vi "Filter.vi"(8 "error in (no error)":errorcluster, 10 "Selected Runnables":string[](array[string]), 11 "LUnit Test Suite In":refnum<class "LUnit Test Suite.lvclass">) -> (0 "error out":errorcluster, 3 "LUnit Test Suite Out":refnum<class "LUnit Test Suite.lvclass">)   [LabVIEW 2020, in "LUnit Test Suite.lvclass"]
doc: "Select which tests are active. This applies recursively to nested suites."
uses:
  LUnit Test Suite.lvclass
  C:/git/astemes-lunit/source/Core/Runnable/Runnable.lvclass
  LUnit Test Suite.lvclass/LUnit Test Suite.ctl
  <vilib>/Utility/miscctls.llb/LVMapReplaceAction.ctl
  Runnable/Runnable.lvclass
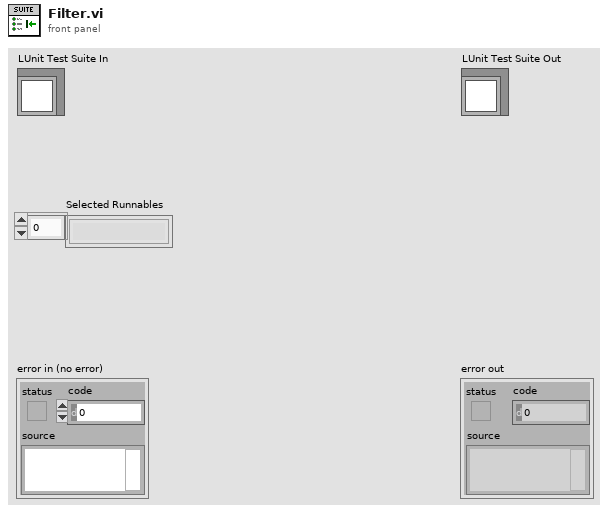
[diagram p1: front panel]
types:
  T1 = typedef "LVMapReplaceAction.ctl" = enum32{"Modify Entry only if found", "Add or Modify Entry", "Delete Entry"}
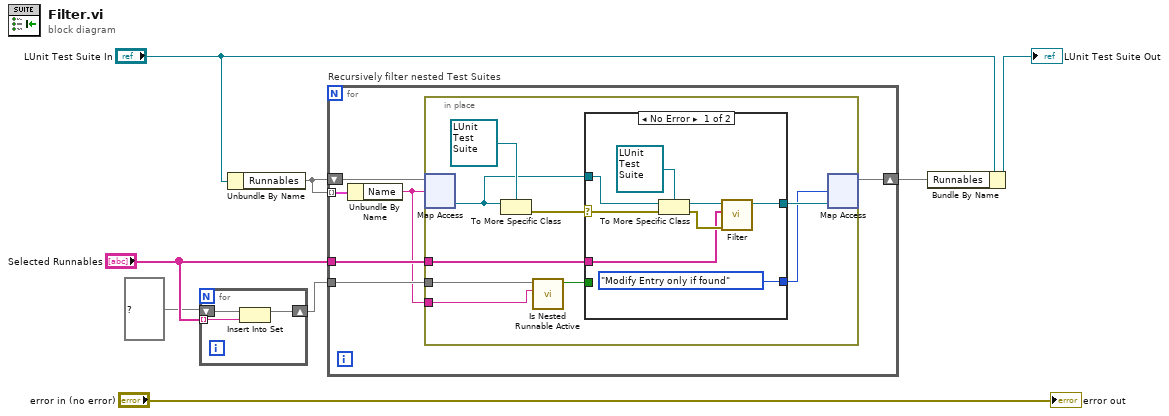
[diagram p0: block diagram]
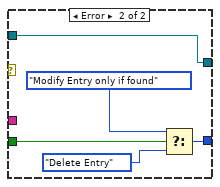
[diagram p2: hidden frame]
diagram:
  n1 = for {
    shift-right: [w10] -> w1
    shift-left: set{string} {} ("set") -> [w11]
    tunnel: "Selected Runnables" -> [w9] mode=indexing
    n2 = Insert Into Set(10:w9, 11:w11) -> (3:w10:set{string})  [unwired: 1 out]
  }
  n3 = Unbundle By Name("LUnit Test Suite In") -> ("Runnables"=w3:map{string, refnum<class "Runnable.lvclass">})
  n4 = for "Recursively filter nested Test Suites" {
    shift-right: [w16] -> w2
    shift-left: w3 -> [w17]
    tunnel: w3 -> [w14] mode=indexing
    tunnel: "Selected Runnables" -> [w15]
    tunnel: w1 -> [w13]
    n5 = Unbundle By Name(w14) -> ("Name"=w12:string)
    n6 = in-place {
      in-place-border: w15 -> [w22]
      in-place-border: w13 -> [w21]
      in-place-border: w12 -> [w20]
      n7 = in-place-map #1(w17, w12) -> (w24:refnum<class "Runnable.lvclass">)  [unwired: 1 in, 1 out]
      n8 = To More Specific Class(target class=refnum<class "LUnit Test Suite.lvclass"> refnum ("LUnit Test Suite V2.lvclass"), reference=w24) -> (error out=w25:errorcluster)  [unwired: 1 in, 1 out]
      n9 = call "Is Nested Runnable Active.vi"("Name"=w20, "Active Methods"=w21) -> ("found?"=w19:bool)  [unwired: 9 in]
      n10 = case shown="No Error" w25 {
        selector: w25 -> [w32 _]
        tunnel: w24 -> [w33 w39]
        tunnel: [w29 w39] -> w23
        tunnel: w22 -> [w28 _]
        tunnel: w19 -> [_ w38]
        tunnel: [LVMapReplaceAction."Modify Entry only if found" ("action") w37] -> w18
        frame No Error {
          n11 = To More Specific Class(target class=refnum<class "LUnit Test Suite.lvclass"> refnum ("LUnit Test Suite V2.lvclass"), reference=w33, error in=w32) -> (specific class reference=w31:refnum<class "LUnit Test Suite.lvclass">, error out=w30:errorcluster)
          n12 = call "Filter.vi"("error in (no error)"=w30, "Selected Runnables"=w28, "LUnit Test Suite In"=w31) -> ("LUnit Test Suite Out"=w29:refnum<class "LUnit Test Suite.lvclass">)  [unwired: 7 in, 1 out]
        }
        frame Error {
          n13 = Select(t=LVMapReplaceAction."Modify Entry only if found" ("action"), s=w38, f=LVMapReplaceAction."Delete Entry" ("action")) -> (s? t:f=w37:T1)
        }
      }
      n14 = in-place-map #1(w23, w18) -> (w16:map{string, refnum<class "Runnable.lvclass">})  [unwired: 2 out]
    }
  }
  n15 = Bundle By Name(cluster="LUnit Test Suite In", "Runnables"=w2) -> (→"LUnit Test Suite Out":refnum<class "LUnit Test Suite.lvclass">)
  "error out" <- "error in (no error)"
